vi "_071.vi"() -> ()   [LabVIEW 2024]
panel:
  out "Boolean 2":bool
  out "Boolean":bool
  out "s? t:f":dbl
  out "element 2":dbl
  out "output array 2":dbl[](array[numeric])
  out "output array":dbl[][](array[numeric])
  out "subarray":dbl[](array[numeric])
  in  "Array":dbl[](array[numeric])
  out "element":dbl
  out "x+y":dbl
  out "Numeric":i32
  # "Logics :"
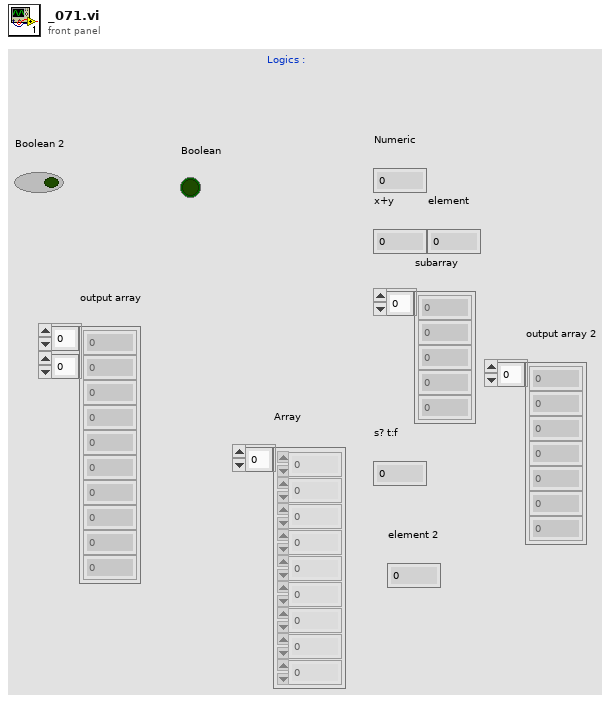
[diagram p1: front panel]
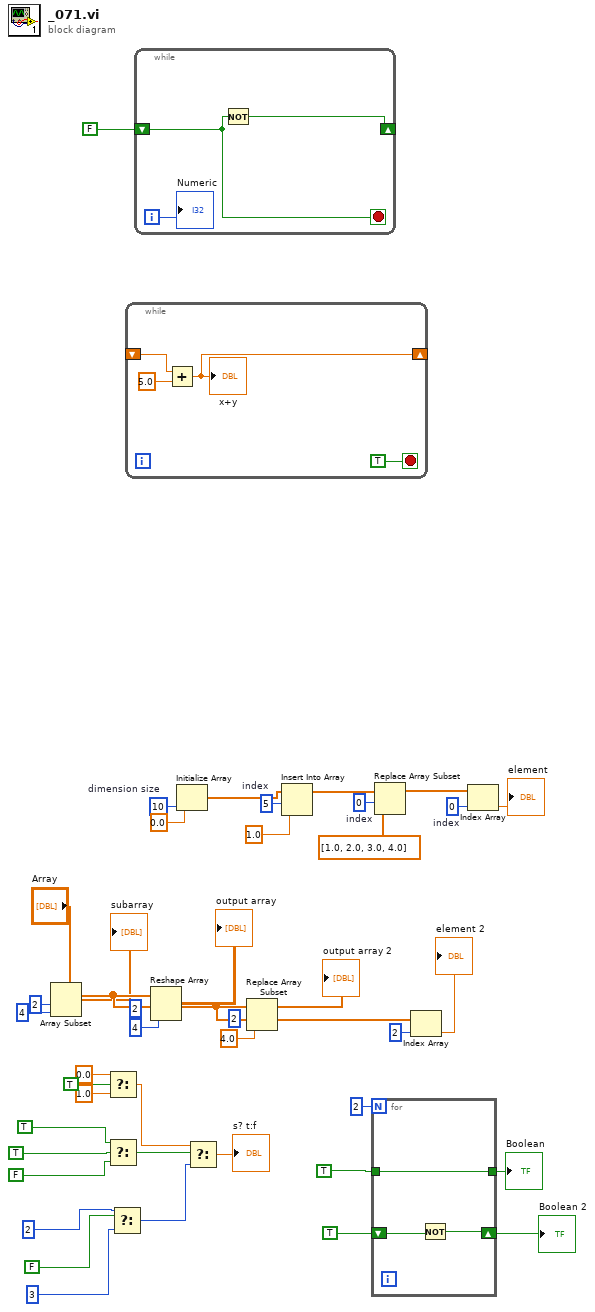
[diagram p0: block diagram]
diagram:
  w38 = 0  # index
  w39 = 0  # index
  w40 = 5  # index
  w41 = 10  # dimension size
  n1 = Array Subset "Array Subset"(array="Array", index=2, length=4) -> (→"subarray":dbl[])
  n2 = Select(t=0.0, s=TRUE, f=1.0) -> (s? t:f=w11:dbl)
  n3 = Select(t=TRUE, s=TRUE, f=FALSE) -> (s? t:f=w12:bool)
  n4 = Select(t=2, s=FALSE, f=3) -> (s? t:f=w7:i32)
  n5 = while {
    shift-right: [w44] -> _
    shift-left: _ -> [w46]
    stop <- TRUE stop-if-true
    n6 = Add(x=w46, y=5.0) -> (x+y=w44:dbl)
    "x+y" <- w44
  }
  n7 = while {
    shift-right: [w47] -> _
    shift-left: FALSE -> [w48]
    i -> [w49]
    stop <- w48 stop-if-true
    n8 = Not(x=w48) -> (.not. x?=w47:bool)
    "Numeric" <- w49
  }
  n9 = Reshape Array "Reshape Array"("Array", 2 ("dimension size"), 4 ("dimension size")) -> (→"output array":dbl[][])
  n10 = Initialize Array "Initialize Array"(0.0 ("element"), w41) -> (w34:dbl[])
  n11 = Select(t=w11, s=w12, f=w7) -> (s? t:f=→"s? t:f":dbl)
  n12 = Replace Array Subset "Replace Array Subset"(array="Array", new element=4.0 ("new element/subarray"), index=2) -> (→"output array 2":dbl[])
  n13 = Insert Into Array "Insert Into Array"(array=w34, index=w40, new element=1.0 ("new element/subarray")) -> (w33:dbl[])
  n14 = for {
    N: 2 -> [_]
    tunnel: TRUE -> [w50]
    shift-right: [w51] -> w1
    shift-left: TRUE -> [w52]
    tunnel: [w50] -> w2
    n15 = Not(x=w52) -> (.not. x?=w51:bool)
  }
  "Boolean" <- w2
  "Boolean 2" <- w1
  n16 = Replace Array Subset "Replace Array Subset"(array=w33, new element=dbl[] [1.0, 2.0, 3.0, 4.0] ("new element/subarray"), index=w39) -> (w32:dbl[])
  n17 = Index Array "Index Array"(array="Array", index=2) -> (element=→"element 2":dbl)
  n18 = Index Array "Index Array"(array=w32, index=w38) -> (element=→"element":dbl)
